vi "Config - supervisory settings.vi"(5 ".ini Controller":enum16{"Read", "Write"}(ring), 7 ".ini filename":string="supervisoryconfig.ini", 8 "error in (no error)":errorcluster, 10 "Supervisory Config Cluster In":T1={"UI Information"={"Header Image"=path "../Data/header.png", "Language"=enum."English", "First Run?"=FALSE, "Setup Camera?"=FALSE, "Device Type"=enum."RCA", "Encoder Type"=enum."Tacho", "Version"=enum."RailMeasurement_CAT", "port"=0, "greyscale"=FALSE, "camera index"=0}, "Test Cluster"={"Operator"="", "Description"="", "Line"="", "Start Position"=450000.0, "Run Length"=31.0, "Sensor A Position"=80000.0, "Rail Side"=FALSE, "Distance Direction"=FALSE, "Path"=path "", "Sensor B Position"=0.0, "Visible Chart Distance"=0.0, "Company"="", "Ref Profile"=""}, "RV-HR Settings Cluster"={"Sensor A Calibration"=0.0, "Integrator Time"=0.0, "Encoder Spacing"=0.0, "Encoder Threshold"=0.0, "Sampling Distance"=0, "Swap Direction?"=FALSE, "Min Walking Speed"=0.0, "Max Walking Speed"=0.0, "Distance Format"=0, "Sensor B Calibration"=0.0, "Tacho Pulses/Rev"=0.0, "Wheel Diameter"=0.0, "Max Short Roughness"=0.0, "Max Long Roughness"=0.0, "Measuring Interval"=0.0, "Measuring Length"=0.0, "Wavelengths"=[], "Device Resolution"=0, "Detect Change in Direction?"=FALSE, "Save Images?"=FALSE, "Image Frequency"=0, "Save Video?"=FALSE, "Image Offset"=0.0, "Start Position at 0m?"=FALSE, "Live Corrug Est.?"=FALSE, "Wavelength Corrug"=0, "Distance Corrug"=0, "Update Corrug"=0}} {"RV-HR Settings Cluster"."Image Frequency" items=["2", "3", "5"]; "RV-HR Settings Cluster"."Device Resolution" items=["0.1 µm", "1 µm", "10 µm"]; "RV-HR Settings Cluster"."Distance Format" items=["kilometres", "miles & chains", "metres", "stations", "miles"]; "RV-HR Settings Cluster"."Sampling Distance" items=["1mm", "2mm"]}, 11 "Directory Path":path) -> (0 "error out":errorcluster, 1 "appended path":path, 2 "Supervisory Config Cluster Out":T1={"UI Information"={"Header Image"=path "../Data/header.png", "Language"=enum."English", "First Run?"=FALSE, "Setup Camera?"=FALSE, "Device Type"=enum."RCA", "Encoder Type"=enum."Tacho", "Version"=enum."RailMeasurement_CAT", "port"=0, "greyscale"=FALSE, "camera index"=0}, "Test Cluster"={"Operator"="", "Description"="", "Line"="", "Start Position"=450000.0, "Run Length"=31.0, "Sensor A Position"=80000.0, "Rail Side"=FALSE, "Distance Direction"=FALSE, "Path"=path "", "Sensor B Position"=0.0, "Visible Chart Distance"=0.0, "Company"="", "Ref Profile"=""}, "RV-HR Settings Cluster"={"Sensor A Calibration"=0.0, "Integrator Time"=0.0, "Encoder Spacing"=0.0, "Encoder Threshold"=0.0, "Sampling Distance"=0, "Swap Direction?"=FALSE, "Min Walking Speed"=0.0, "Max Walking Speed"=0.0, "Distance Format"=0, "Sensor B Calibration"=0.0, "Tacho Pulses/Rev"=0.0, "Wheel Diameter"=0.0, "Max Short Roughness"=0.0, "Max Long Roughness"=0.0, "Measuring Interval"=0.0, "Measuring Length"=0.0, "Wavelengths"=[], "Device Resolution"=0, "Detect Change in Direction?"=FALSE, "Save Images?"=FALSE, "Image Frequency"=0, "Save Video?"=FALSE, "Image Offset"=0.0, "Start Position at 0m?"=FALSE, "Live Corrug Est.?"=FALSE, "Wavelength Corrug"=0, "Distance Corrug"=0, "Update Corrug"=0}} {"RV-HR Settings Cluster"."Image Frequency" items=["2", "3", "5"]; "RV-HR Settings Cluster"."Device Resolution" items=["0.1 µm", "1 µm", "10 µm"]; "RV-HR Settings Cluster"."Distance Format" items=["kilometres", "miles & chains", "metres", "stations", "miles"]; "RV-HR Settings Cluster"."Sampling Distance" items=["1mm", "2mm"]})   [LabVIEW 2023]
doc: "Obtains default hlc configuration information from an .ini file"
uses:
  <vilib>/Utility/config.llb/NI_LVConfig.lvlib
  Controls/UI Init Config Info.ctl
  Controls/Supervisory Config Cluster.ctl
  Controls/Test Cluster.ctl
  Controls/Distance Units.ctl
  Controls/Settings Cluster.ctl
  Controls/Sampling DIstance.ctl
  Controls/Language.ctl
  Controls/Device_Type.ctl
  Controls/EncoderType.ctl
  Controls/Device_Resolution.ctl
  Controls/Software Version.ctl
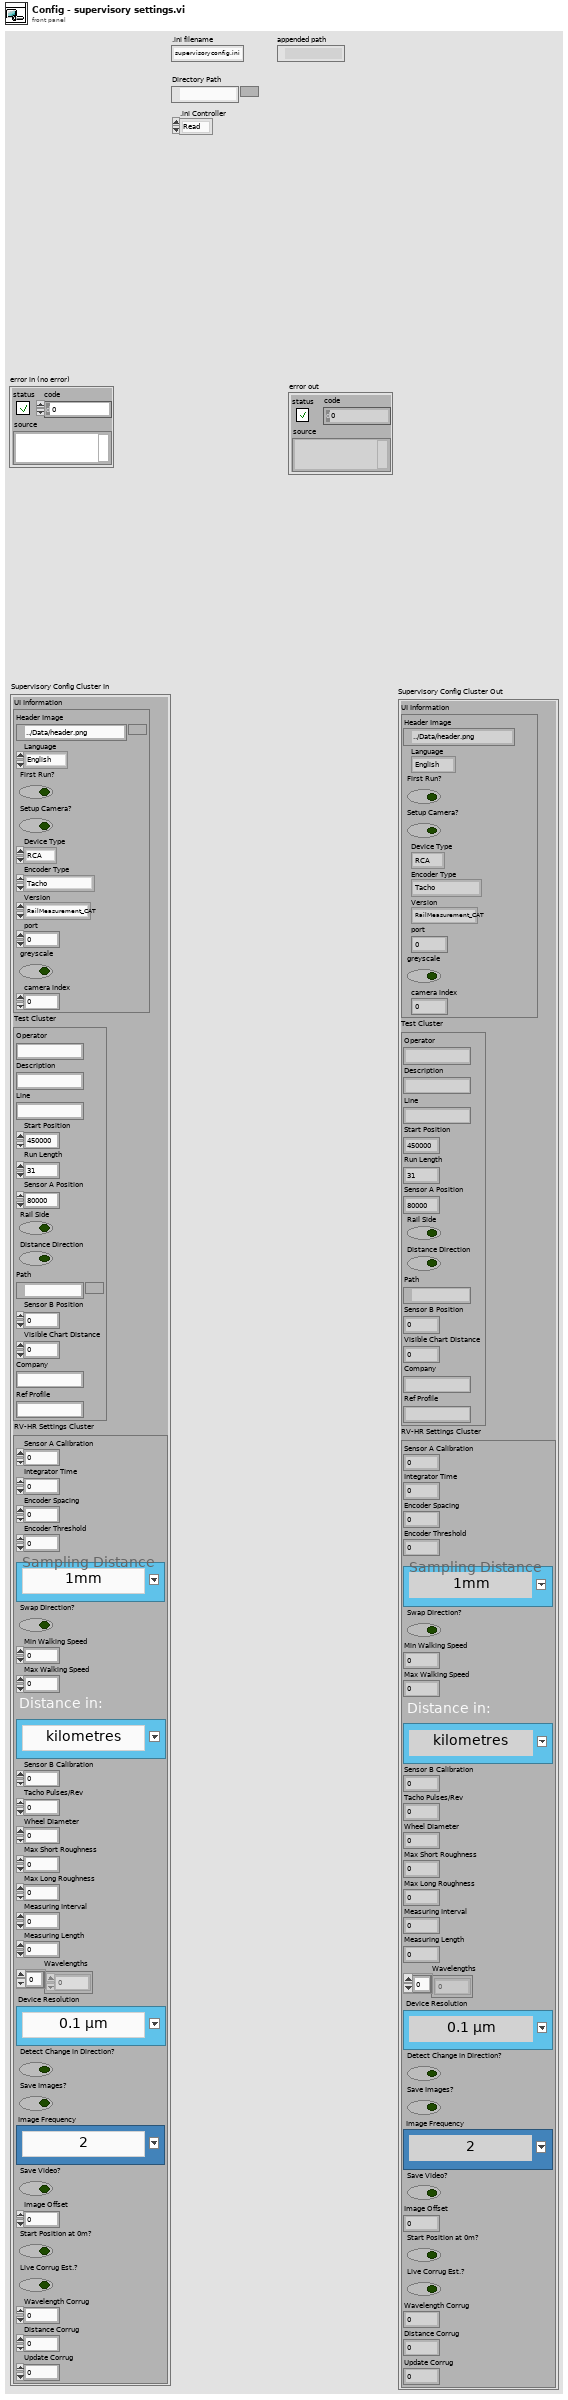
[diagram p1: front panel]
types:
  T1 = typedef "Supervisory Config Cluster.ctl" = cluster{"UI Information":T2, "Test Cluster":T7, "RV-HR Settings Cluster":T8}
  T2 = typedef "UI Init Config Info.ctl" = cluster{"Header Image":path, "Language":T3, "First Run?":bool, "Setup Camera?":bool, "Device Type":T4, "Encoder Type":T5, "Version":T6, "port":i32, "greyscale":bool, "camera index":i32}
  T3 = typedef "Language.ctl" = enum16{"English", "Chinese", "German"}
  T4 = typedef "Device_Type.ctl" = enum16{"CAT", "Bi-CAT", "YRCA", "RCA", "RV-HR", "TV-HR"}
  T5 = typedef "EncoderType.ctl" = enum16{"Tacho", "Quadrature"}
  T6 = typedef "Software Version.ctl" = enum16{"RailMeasurement_CAT", "RailMeasurement_Master", "RailMeasurement_RCA", "RailMeasurement_CAT-V", "RailMeasurement_RCA-V", "RailMeasurement_RV-HR"}
  T7 = typedef "Test Cluster.ctl" = cluster{"Operator":string, "Description":string, "Line":string, "Start Position":dbl, "Run Length":dbl, "Sensor A Position":dbl, "Rail Side":bool, "Distance Direction":bool, "Path":path, "Sensor B Position":dbl, "Visible Chart Distance":dbl, "Company":string, "Ref Profile":string}
  T8 = typedef "Settings Cluster.ctl" = cluster{"Sensor A Calibration":dbl, "Integrator Time":dbl, "Encoder Spacing":dbl, "Encoder Threshold":dbl, "Sampling Distance":T9, "Swap Direction?":bool, "Min Walking Speed":dbl, "Max Walking Speed":dbl, "Distance Format":T10, "Sensor B Calibration":dbl, "Tacho Pulses/Rev":dbl, "Wheel Diameter":dbl, "Max Short Roughness":dbl, "Max Long Roughness":dbl, "Measuring Interval":dbl, "Measuring Length":dbl, "Wavelengths":dbl[], "Device Resolution":T11, "Detect Change in Direction?":bool, "Save Images?":bool, "Image Frequency":T9, "Save Video?":bool, "Image Offset":dbl, "Start Position at 0m?":bool, "Live Corrug Est.?":bool, "Wavelength Corrug":u8, "Distance Corrug":u8, "Update Corrug":u8}
  T9 = typedef "Sampling DIstance.ctl" = u16
  T10 = typedef "Distance Units.ctl" = u16
  T11 = typedef "Device_Resolution.ctl" = u16
  T12 = typedef "NI_LVConfig.lvlib/Config Data RefNum.ctl" = refnum<k1>
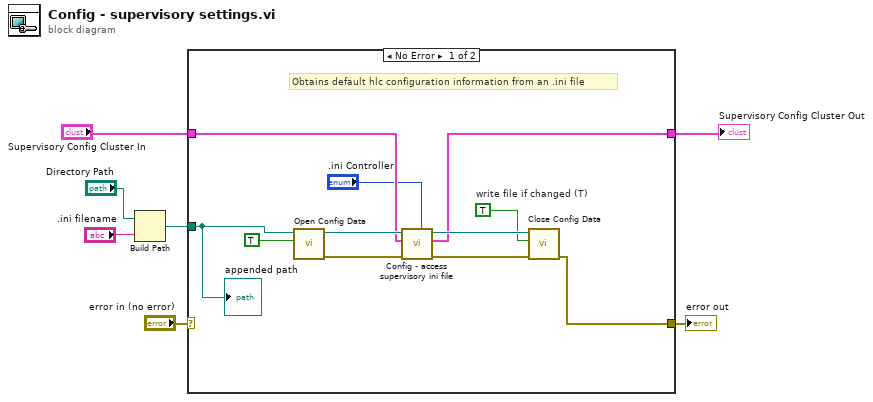
[diagram p0: block diagram]
diagram:
  n1 = Build Path(base path="Directory Path", name or relative path=".ini filename") -> (appended path=w5:path)
  n2 = case shown="No Error" "error in (no error)" {
    selector: "error in (no error)" -> [_ w19]
    tunnel: [w12 _] -> w1
    tunnel: [w11 w19] -> w6
    tunnel: w5 -> [w10 _]
    tunnel: "Supervisory Config Cluster In" -> [w9 _]
    frame No Error {
      w14 = TRUE  # write file if changed (T)
      # "Obtains default hlc configuration information from an .ini file"
      n3 = call <vilib>:"Open Config Data.vi"("create file if necessary (T)"=TRUE, "configuration file path"=w10) -> ("error out"=w17:errorcluster, "refnum"=w15:T12)  [unwired: 7 in, 1 out]
      n4 = call "Config - access supervisory ini file.vi"(".ini Controller"=".ini Controller", "error in"=w17, "HLC Controls"=w9, "Config File Ref"=w15) -> ("error out"=w18:errorcluster, "HLC Controls Out"=w12:T1, "refnum out"=w16:T12)  [unwired: 5 in]
      n5 = call <vilib>:"Close Config Data.vi"("error in (no error)"=w18, "write file if changed (T)"=w14, "refnum"=w16) -> ("error out"=w11:errorcluster)  [unwired: 7 in, 1 out]
      "appended path" <- w10
    }
    frame Error {
    }
  }
  "error out" <- w6
  "Supervisory Config Cluster Out" <- w1
